vi "SP Find Next Waveform Name.vi"(8 "error in (no error)":errorcluster, 9 "Prospective Base Name":string, 10 "Attribute Name (NI_ChannelName)":string, 11 "Waveforms in":waveform(dbl)[](array[waveform])) -> (0 "error out":errorcluster, 1 "Channel Name":string)   [LabVIEW 2011]
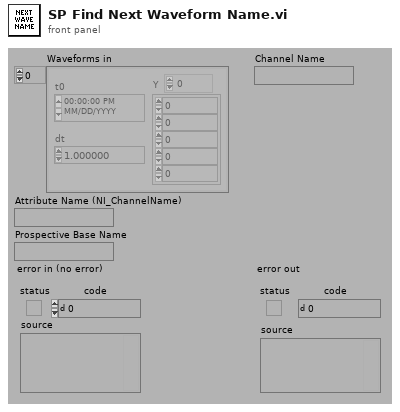
[diagram p1: front panel]
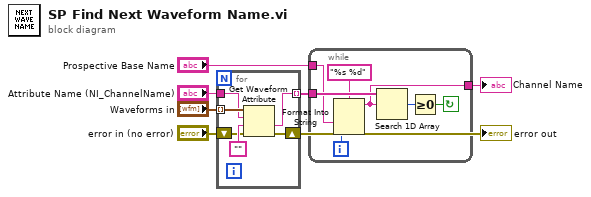
[diagram p0: block diagram]
diagram:
  n1 = for {
    tunnel: "Waveforms in" -> [w13] mode=indexing
    tunnel: "Attribute Name (NI_ChannelName)" -> [w11]
    shift-right: [w9] -> w4
    shift-left: "error in (no error)" -> [w10]
    tunnel: [w8] -> w2 mode=indexing
    n2 = Get Waveform Attribute(4:w10, 5:"", 6:w11, 7:w13) -> (0:w9:errorcluster, 1:w8:string)  [unwired: 2 out]
  }
  "error out" <- w4
  n3 = while {
    tunnel: "Prospective Base Name" -> [w16]
    tunnel: w2 -> [w20]
    tunnel: [w14] -> w1
    i -> [w15]
    stop <- w18 continue-if-true
    n4 = Format Into String(format string="%s %d", w16, w15) -> (resulting string=w14:string)  [unwired: 2 in, 1 out]
    n5 = Search 1D Array(1D array=w20, element=w14) -> (index of element=w19:i32)  [unwired: 1 in]
    n6 = Greater Or Equal To 0?(x=w19) -> (x >= 0?=w18:bool)
  }
  "Channel Name" <- w1
